vi "Mark as Source Only.vi"() -> ()   [LabVIEW 2014]
panel:
  out "Progess":i32(slide) scale=0.0..2947.0
  in  "Mark VIs":bool
  in  "IgnoreSVN":bool
  in  "Root Folder":path
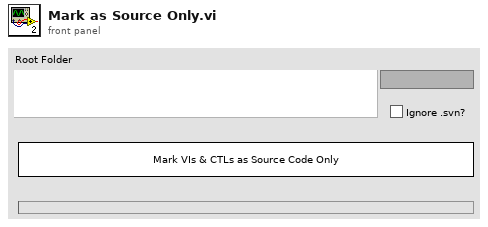
[diagram p1: front panel]
types:
  T1 = enum32{"invalid VI type", "Standard VI", "Control VI", "Global VI", "Polymorphic VI", "Configuration VI", "SubSystem", "Facade VI", "Method VI", "Statechart Diagram VI"}[]
  T2 = enum32{"invalid VI type", "Standard VI", "Control VI", "Global VI", "Polymorphic VI", "Configuration VI", "SubSystem", "Facade VI", "Method VI", "Statechart Diagram VI"}
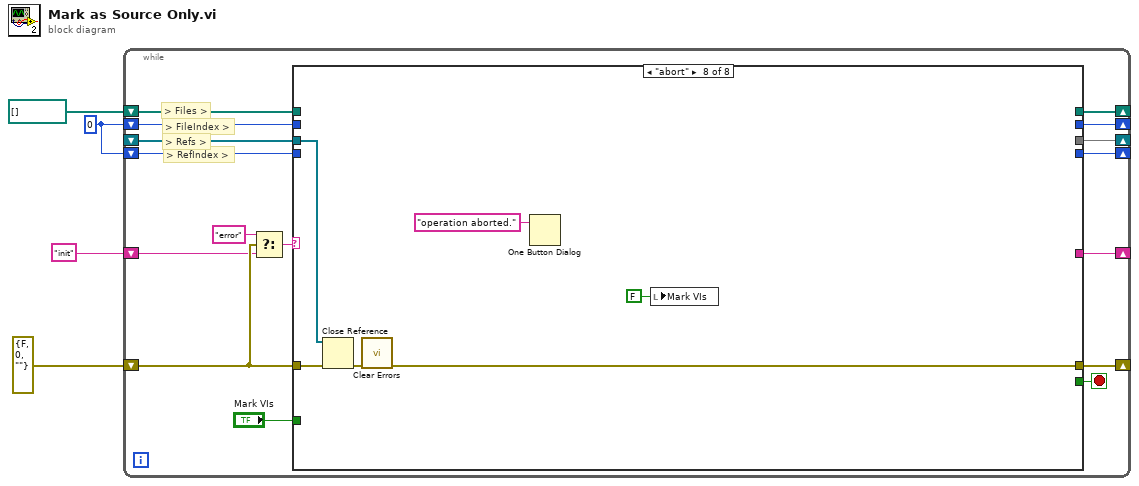
[diagram p0: block diagram]
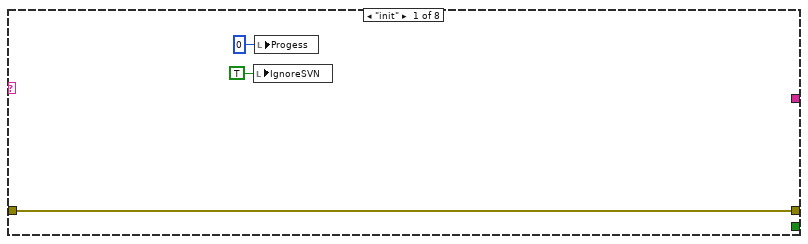
[diagram p2: hidden frame]
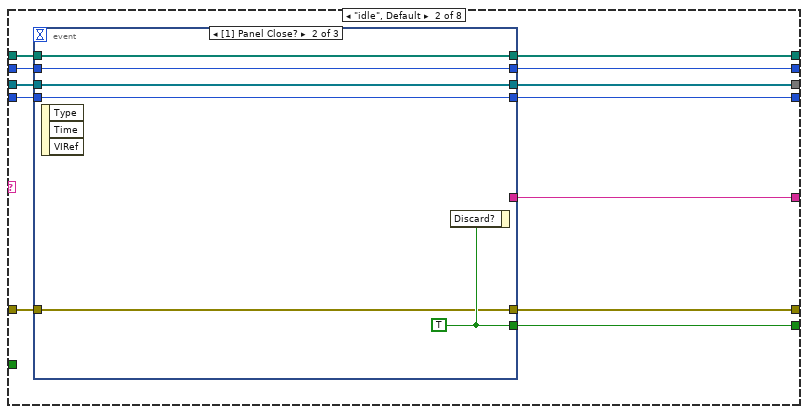
[diagram p3: hidden frame]
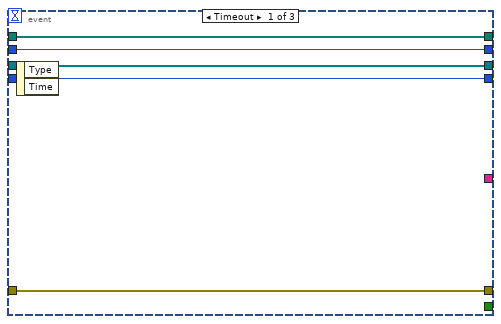
[diagram p4: hidden frame]
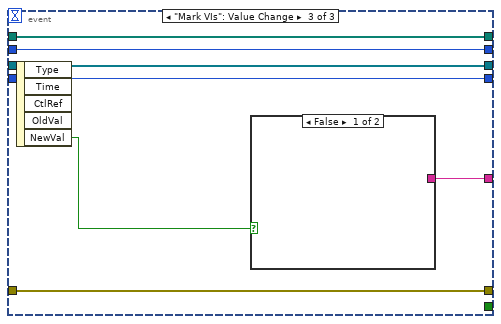
[diagram p5: hidden frame]
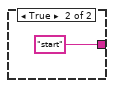
[diagram p6: hidden frame]
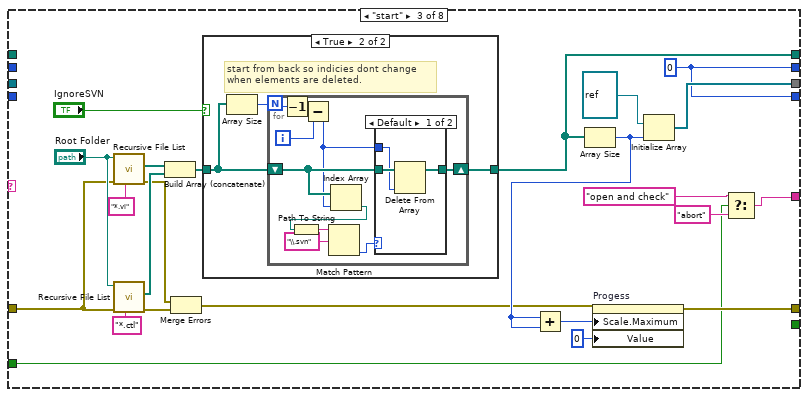
[diagram p7: hidden frame]
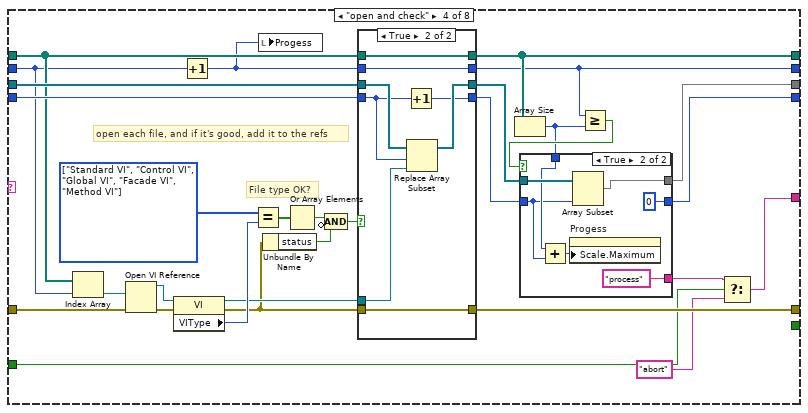
[diagram p10: hidden frame]
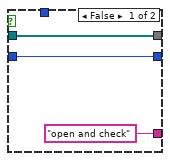
[diagram p11: hidden frame]
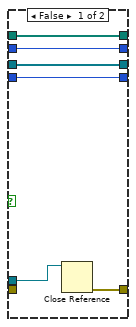
[diagram p12: hidden frame]
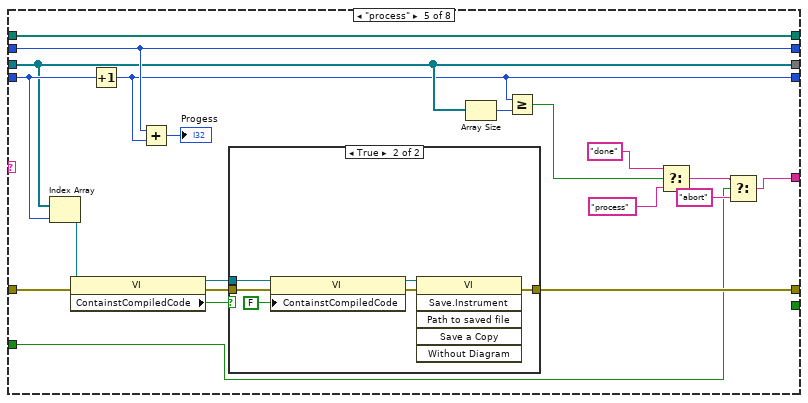
[diagram p13: hidden frame]
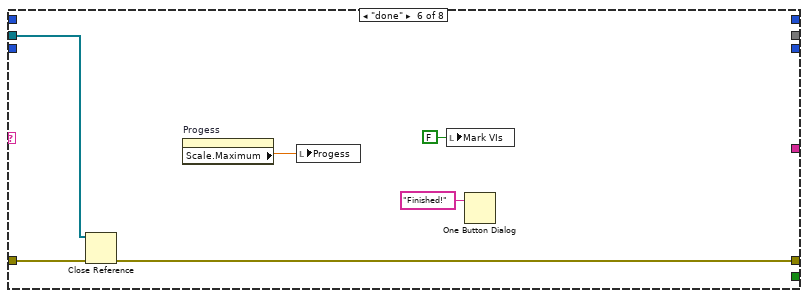
[diagram p15: hidden frame]
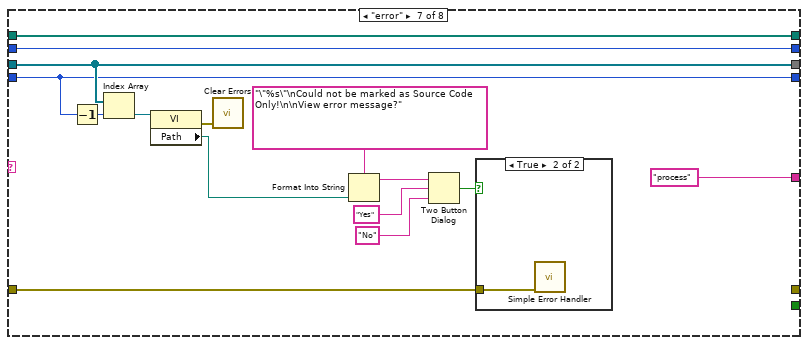
[diagram p16: hidden frame]
diagram:
  w1 = 0
  n1 = while {
    shift-right: [w15] -> _
    shift-left: "init" -> [w6]
    shift-right: [w16] -> _
    shift-left: errorcluster {"status"=FALSE, "code"=0, "source"=""} ("error in") -> [w17]
    shift-right: [w14] -> _
    shift-left: path[] [] -> [w13]
    shift-right: [w11] -> _
    shift-left: w1 -> [w12]
    shift-right: [w10] -> _
    shift-left: _ -> [w9]
    shift-right: [w7] -> _
    shift-left: w1 -> [w8]
    stop <- w20 stop-if-true
    # "> RefIndex >"
    # "> Refs >"
    # "> FileIndex >"
    # "> Files >"
    n2 = Select(t="error", s=w17, f=w6) -> (s? t:f=w18:string)
    n3 = case shown="\"abort\"" w18 {
      tunnel: [_ w35 _ _ _ _ _ _] -> w20
      tunnel: w17 -> [w23 w34 w63 w125 w165 w182 w185 w201]
      tunnel: [w23 w33 w72 w111 w160 w180 _ w199] -> w16
      tunnel: [_ w32 w56 w97 w152 _ "process" _] -> w15
      tunnel: [_ w29 w59 w108 w166 _ w197 _] -> w14
      tunnel: w13 -> [_ w31 _ w112 w166 _ w197 _]
      tunnel: w12 -> [_ w30 _ w109 w167 _ w196 _]
      tunnel: [_ w28 w66 w104 w167 _ w196 _] -> w11
      tunnel: [_ w27 w69 w102 w159 _ w194 _] -> w10
      tunnel: w9 -> [_ w26 _ w118 w159 w181 w194 w202]
      tunnel: w8 -> [_ w25 _ w116 w169 _ w192 _]
      tunnel: [_ w24 w66 w105 w157 _ w192 _] -> w7
      tunnel: "Mark VIs" -> [_ _ w55 w99 w150 _ _ _]
      frame "init" {
        n4 = local write "IgnoreSVN"(TRUE ("IgnoreSVN")) -> ()
        n5 = local write "Progess"(0 ("Progess")) -> ()
      }
      frame "idle", Default {
        n6 = event shown="[1] Panel Close?" {
          selector: _ -> [_ _ _]
          dyn-events: _ -> [_ _ _]
          timeout: _ -> [_ _ _]
          tunnel: [_ w46 _] -> w35
          tunnel: w34 -> [w40 w45 w53]
          tunnel: [w40 w45 w53] -> w33
          tunnel: [_ _ w52] -> w32
          tunnel: w31 -> [w38 w44 w50]
          tunnel: w30 -> [w39 w43 w51]
          tunnel: [w38 w44 w50] -> w29
          tunnel: [w39 w43 w51] -> w28
          tunnel: [w36 w42 w48] -> w27
          tunnel: w26 -> [w36 w42 w48]
          tunnel: w25 -> [w37 w41 w49]
          tunnel: [w37 w41 w49] -> w24
          event Timeout {
            n7 = event-data() -> ()  [unwired: 1 in, 2 out]
          }
          event Panel Close? {
            w46 = TRUE
            n8 = event-data() -> ()  [unwired: 1 in, 3 out]
            n9 = event-data("Discard?"=w46) -> ()  [unwired: 1 in, 1 out]
          }
          event "Mark VIs": Value Change {
            n10 = event-data() -> ("NewVal"=w47:bool)  [unwired: 1 in, 4 out]
            n11 = case shown="False" w47 {
              tunnel: [_ "start"] -> w52
              frame False {
              }
              frame True {
              }
            }
          }
        }
      }
      frame "start" {
        w66 = 0
        n12 = call <vilib>:"Recursive File List.vi"("pattern"="*.vi", "error in (no error)"=w63, "Folder Path"="Root Folder") -> ("error out"=w64:errorcluster, "All Files in Dir"=w74:path[])  [unwired: 4 in, 3 out]
        n13 = call <vilib>:"Recursive File List.vi"("pattern"="*.ctl", "error in (no error)"=w63, "Folder Path"="Root Folder") -> ("error out"=w62:errorcluster, "All Files in Dir"=w73:path[])  [unwired: 4 in, 3 out]
        n14 = Build Array (concatenate)(w74, w73) -> (w65:path[])
        n15 = Merge Errors(w64, w62) -> (w61:errorcluster)
        n16 = case shown="True" "IgnoreSVN" {
          tunnel: w65 -> [w78 w79]
          tunnel: [w78 w81] -> w59
          frame False {
          }
          frame True {
            # "start from back so indicies dont change\nwhen elements are deleted."
            n17 = Array Size(array=w79) -> (size(s)=w80:i32)
            n18 = for {
              N: w80 -> [w91]
              shift-right: [w83] -> w81
              shift-left: w79 -> [w86]
              i -> [w90]
              n19 = Decrement(x=w91) -> (x-1=w82:i32)
              n20 = Subtract(x=w82, y=w90) -> (x-y=w85:i32)
              n21 = Index Array(array=w86, index=w85) -> (element=w89:path)
              n22 = Path To String(path=w89) -> (string=w88:string)
              n23 = Match Pattern(string=w88, regular expression="\\.svn") -> (offset past match=w84:i32)  [unwired: 1 in, 3 out]
              n24 = case shown="Default" w84 {
                tunnel: w86 -> [w94 w95]
                tunnel: w85 -> [w92 _]
                tunnel: [w93 w95] -> w83
                frame Default {
                  n25 = Delete From Array(array=w94, index=w92) -> (array with subset deleted=w93:path[])  [unwired: 1 in, 1 out]
                }
                frame -1 {
                }
              }
            }
          }
        }
        n26 = Array Size(array=w59) -> (size(s)=w67:i32)
        n27 = Add(x=w67, y=w67) -> (x+y=w68:i32)
        n28 = property on="Progess" class="Slide (strict)"(error in=w61, "Scale.Maximum"=w68, "Value"=0 ("Progess")) -> (error out=w72:errorcluster)  [unwired: 1 in, 1 out]
        n29 = Initialize Array(refnum<vi> refnum ("This VI"), w67) -> (w69:refnum<vi>[])
        n30 = Select(t="open and check", s=w55, f="abort") -> (s? t:f=w56:string)
      }
      frame "open and check" {
        w120 = T1 [enum."Standard VI", enum."Control VI", enum."Global VI", enum."Facade VI", enum."Method VI"] items=["invalid VI type", "Standard VI", "Control VI", "Global VI", "Polymorphic VI", "Configuration VI", "SubSystem", "Facade VI", "Method VI", "Statechart Diagram VI"]
        # "open each file, and if it's good, add it to the refs"
        # "File type OK?"
        n31 = Index Array(array=w112, index=w109) -> (element=w124:path)
        n32 = Open VI Reference(vi path=w124, error in (no error)=w125) -> (vi reference=w122:refnum<vi>, error out=w123:errorcluster)  [unwired: 4 in]
        n33 = property class="VI"(reference=w122, error in=w123) -> (reference out=w117:refnum<vi>, error out=w110:errorcluster, "VIType"=w121:T2)
        n34 = Increment(x=w109) -> (x+1=w103:i32)
        n35 = Equal?(x=w120, y=w121) -> (x = y?=w119:bool[])
        n36 = local write "Progess"(w103) -> ()
        n37 = Unbundle By Name(w110) -> ("status"=w114:bool)
        n38 = Or Array Elements(Boolean array=w119) -> (logical OR=w115:bool)
        n39 = Compound Arithmetic op=AND(w115, invert w114) -> (w113:bool)
        n40 = case shown="True" w113 {
          tunnel: w118 -> [w139 w149]
          tunnel: w117 -> [w137 w148]
          tunnel: [w139 w147] -> w106
          tunnel: w116 -> [w138 w146]
          tunnel: [w138 w145] -> w101
          tunnel: w112 -> [w141 w144]
          tunnel: [w141 w144] -> w108
          tunnel: [w140 w143] -> w104
          tunnel: w103 -> [w140 w143]
          tunnel: [w136 w142] -> w111
          tunnel: w110 -> [_ w142]
          frame False {
            n41 = Close Reference(reference=w137) -> (error out=w136:errorcluster)  [unwired: 1 in]
          }
          frame True {
            n42 = Increment(x=w146) -> (x+1=w145:i32)
            n43 = Replace Array Subset(array=w149, new element=w148, index=w146) -> (w147:refnum<vi>[])
          }
        }
        n44 = Array Size(array=w108) -> (size(s)=w100:i32)
        n45 = Greater Or Equal?(x=w104, y=w100) -> (x >= y?=w107:bool)
        n46 = case shown="True" w107 {
          tunnel: w106 -> [w128 w133]
          tunnel: w101 -> [w127 w129]
          tunnel: [w128 w132] -> w102
          tunnel: [w127 0] -> w105
          tunnel: ["open and check" "process"] -> w96
          tunnel: w100 -> [_ w130]
          frame False {
          }
          frame True {
            n47 = Add(x=w130, y=w129) -> (x+y=w134:i32)
            n48 = property on="Progess" class="Slide (strict)"("Scale.Maximum"=w134) -> ()  [unwired: 2 in, 2 out]
            n49 = Array Subset(array=w133, length=w129) -> (w132:refnum<vi>[])  [unwired: 1 in]
          }
        }
        n50 = Select(t=w96, s=w99, f="abort") -> (s? t:f=w97:string)
      }
      frame "process" {
        n51 = Index Array(array=w159, index=w169) -> (element=w164:refnum<vi>)
        n52 = property class="VI"(reference=w164, error in=w165) -> (reference out=w163:refnum<vi>, error out=w162:errorcluster, "ContainstCompiledCode"=w161:bool)
        n53 = Increment(x=w169) -> (x+1=w157:i32)
        n54 = Add(x=w167, y=w157) -> (x+y=→"Progess":i32)
        n55 = case shown="True" w161 {
          tunnel: w163 -> [_ w176]
          tunnel: w162 -> [w170 w175]
          tunnel: [w170 w171] -> w160
          frame False {
            # "no change needed - compiled code\nnot present."
          }
          frame True {
            n56 = property class="VI"(reference=w176, error in=w175, "ContainstCompiledCode"=FALSE ("Contains Compiled Code")) -> (reference out=w172:refnum<vi>, error out=w173:errorcluster)
            n57 = invoke class="VI" method="Save.Instrument"(reference=w172, error in=w173) -> (error out=w171:errorcluster)  [unwired: 4 in, 5 out]
          }
        }
        n58 = Array Size(array=w159) -> (size(s)=w158:i32)
        n59 = Greater Or Equal?(x=w157, y=w158) -> (x >= y?=w156:bool)
        n60 = Select(t="done", s=w156, f="process") -> (s? t:f=w153:string)
        n61 = Select(t=w153, s=w150, f="abort") -> (s? t:f=w152:string)
      }
      frame "done" {
        n62 = Close Reference(reference=w181, error in (no error)=w182) -> (error out=w180:errorcluster)
        n63 = property on="Progess" class="Slide (strict)"() -> ("Scale.Maximum"=w179:dbl)  [unwired: 2 in, 2 out]
        n64 = local write "Progess"(w179) -> ()
        n65 = local write "Mark VIs"(FALSE ("Mark VIs")) -> ()
        n66 = One Button Dialog(message="Finished!") -> ()  [unwired: 1 in, 1 out]
      }
      frame "error" {
        n67 = Decrement(x=w192) -> (x-1=w193:i32)
        n68 = Index Array(array=w194, index=w193) -> (element=w195:refnum<vi>)
        n69 = property class="VI"(reference=w195) -> (error out=w183:errorcluster, "Path"=w191:path)  [unwired: 1 in, 1 out]
        n70 = call <vilib>:"Clear Errors.vi"("error in (no error)"=w183) -> ()  [unwired: 5 in, 2 out]
        n71 = Format Into String(format string="\"%s\"\nCould not be marked as Source Code Only!\n\nView error message?", w191) -> (resulting string=w189:string)  [unwired: 2 in, 1 out]
        n72 = Two Button Dialog(message=w189, 1:"No" ("F button name (\"Cancel\")"), 2:"Yes" ("T button name (\"OK\")")) -> (T button?=w186:bool)
        n73 = case shown="True" w186 {
          tunnel: w185 -> [_ w198]
          frame False {
          }
          frame True {
            n74 = call <vilib>:"Simple Error Handler.vi"("error in (no error)"=w198) -> ()  [unwired: 4 in, 5 out]
          }
        }
      }
      frame "abort" {
        n75 = Close Reference(reference=w202, error in (no error)=w201) -> (error out=w200:errorcluster)
        n76 = call <vilib>:"Clear Errors.vi"("error in (no error)"=w200) -> ("error out"=w199:errorcluster)  [unwired: 5 in, 1 out]
        n77 = One Button Dialog(message="operation aborted.") -> ()  [unwired: 1 in, 1 out]
        n78 = local write "Mark VIs"(FALSE ("Mark VIs")) -> ()
      }
    }
  }
